vi "WhichValvesOpen.vi"(11 "Valves":bool[][](array[boolean])=[[FALSE, FALSE, FALSE], [FALSE, FALSE, FALSE], [FALSE, FALSE, FALSE], [FALSE, FALSE, FALSE], [FALSE, FALSE, FALSE], [FALSE, FALSE, FALSE], [FALSE, FALSE, FALSE], [FALSE, FALSE, FALSE]]) -> (3 "appended array":string[](array[string]))   [LabVIEW 2016]
panel:
  in  "Flowboard":enum16{"A", "B", "C"}(ring)
  in  "Channel":enum16{"1", "2", "3", "4", "5", "6", "7", "8"}(ring)
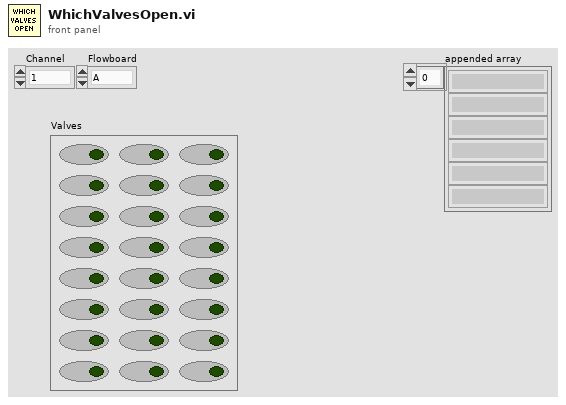
[diagram p1: front panel]
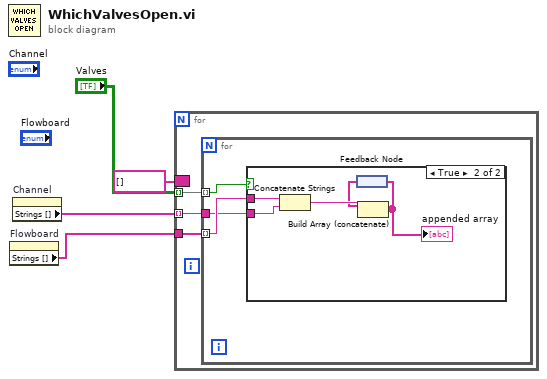
[diagram p0: block diagram]
diagram:
  n1 = property on="Flowboard" class="Enum (strict)"() -> ("Strings []"=w2:string[])  [unwired: 2 in, 2 out]
  n2 = property on="Channel" class="Enum (strict)"() -> ("Strings []"=w3:string[])  [unwired: 2 in, 2 out]
  n3 = for {
    tunnel: "Valves" -> [w7] mode=indexing
    tunnel: w3 -> [w6] mode=indexing
    tunnel: w2 -> [w5]
    border: string[] [] -> [_]
    n4 = for {
      tunnel: w7 -> [w10] mode=indexing
      tunnel: w6 -> [w8]
      tunnel: w5 -> [w9] mode=indexing
      n5 = case shown="True" w10 {
        tunnel: w9 -> [_ w15]
        tunnel: w8 -> [_ w14]
        frame False {
        }
        frame True {
          n6 = Concatenate Strings(w15, w14) -> (w13:string)
          n7 = feedback #1() -> (w11:string[])
          n8 = Build Array (concatenate)(w11, w13) -> (w12:string[])
          "appended array" <- w12
          n9 = feedback-in #1(w12) -> ()
        }
      }
    }
  }
